vi "REPORT_AUDIT_control_index.vi"(7 "option":T1, 10 "array_input":string[][](array[string]), 11 "add_value":i32) -> (2 "array_output":string[][](array[string]), 3 "index_output":i32)   [LabVIEW 2020]
uses:
  typedef/REPORT_AUDIT_control_index.ctl
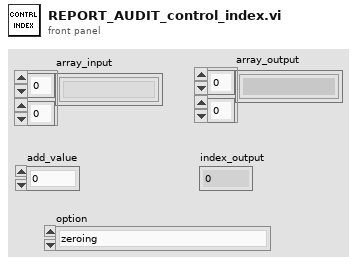
[diagram p1: front panel]
types:
  T1 = typedef "REPORT_AUDIT_control_index.ctl" = enum16{"zeroing", "add_to_index", "get_index"}
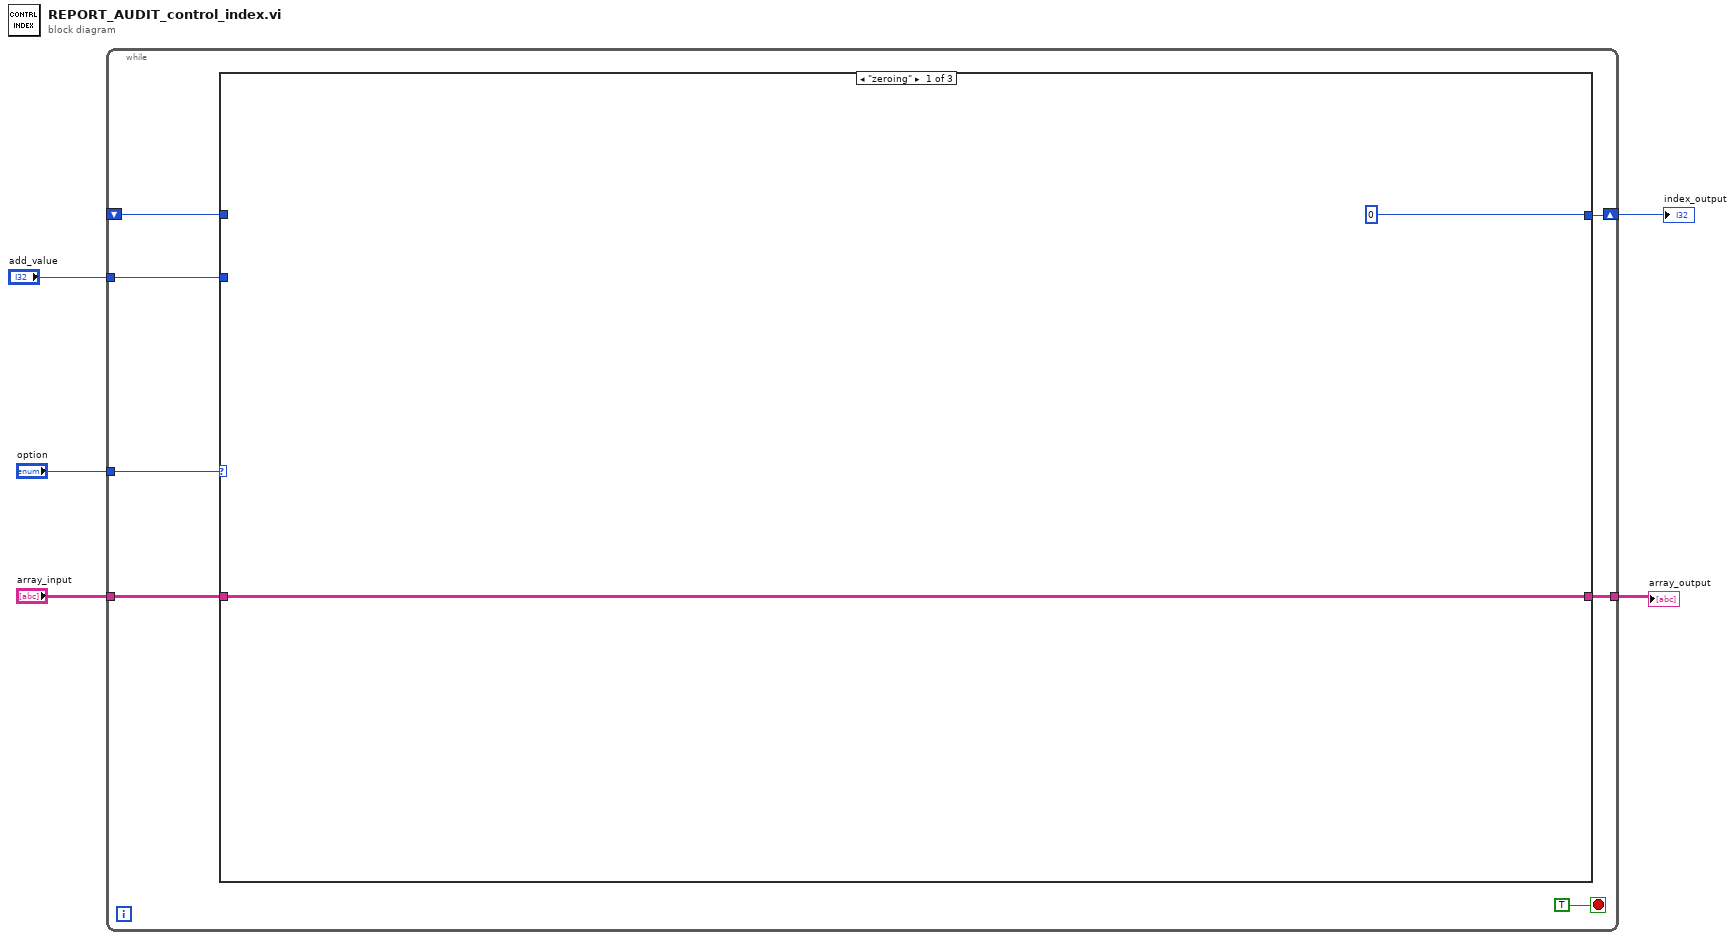
[diagram p0: block diagram]
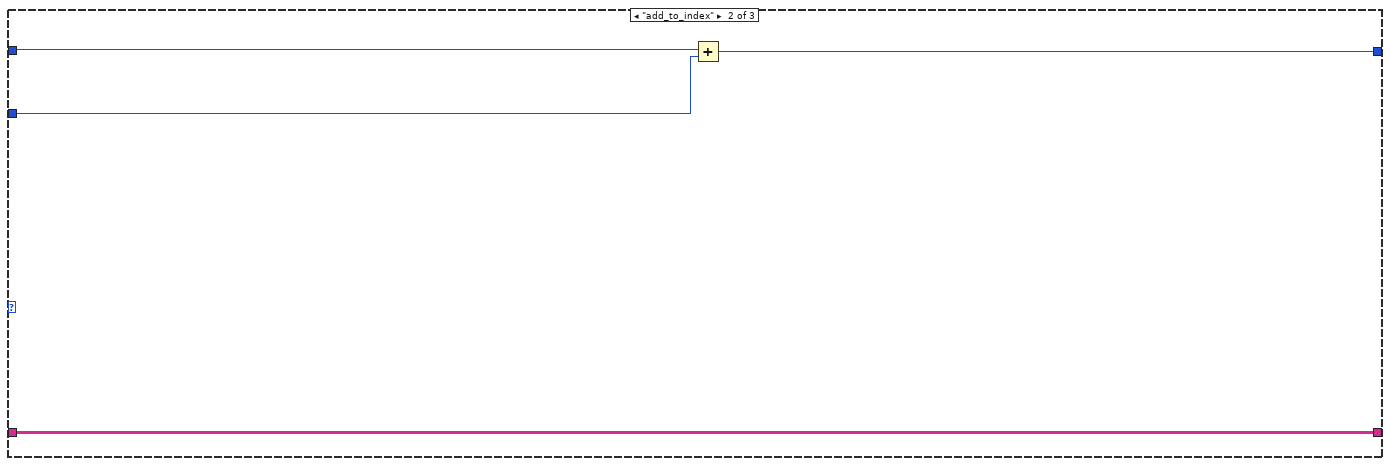
[diagram p2: hidden frame]
diagram:
  n1 = while {
    tunnel: "option" -> [w11]
    shift-right: [w8] -> w4
    shift-left: _ -> [w9]
    tunnel: "add_value" -> [w10]
    tunnel: "array_input" -> [w7]
    tunnel: [w6] -> w1
    stop <- TRUE stop-if-true
    n2 = case shown="\"zeroing\"" w11 {
      tunnel: w10 -> [_ w17 _]
      tunnel: w9 -> [_ w18 w20]
      tunnel: [0 w16 w20] -> w8
      tunnel: w7 -> [w13 w15 w19]
      tunnel: [w13 w15 w19] -> w6
      frame "zeroing" {
      }
      frame "add_to_index" {
        n3 = Add(x=w18, y=w17) -> (x+y=w16:i32)
      }
      frame "get_index" {
      }
    }
  }
  "index_output" <- w4
  "array_output" <- w1
